vi "Pack Subscription Request.vi"(8 "error in (no error)":errorcluster, 9 "Subscription Policy":T1, 10 "Type":variant, 11 "Datum Name":string) -> (0 "error out":errorcluster, 3 "SubscriptionRequest":refnum<class "SubscriptionRequest.lvclass">)   [LabVIEW 2017, in "IMediator.lvlib" / "SubscriptionRequest.lvclass"]
doc: "<License>\nCopyright © 2017 Composed Systems, LLC | All rights reserved\nwww.composed.io\n\nAuthor: Ethan Stern <ethan.stern@composed.io>\n\nThis software is provided \"AS IS\" WITHOUT WARRANTIES, either express or implied, AND IS FOR EDUCATIONAL PURPOSES ONLY.\n</License>"
uses:
  <vilib>/gpm_packages/@cs/mva-core/Source/IMediator/SubscriptionRequest/SubscriptionRequest.lvclass
  <vilib>/gpm_packages/@cs/mva-core/Source/IMediator/ISubscriptionPolicy/ISubscriptionPolicy Reference.ctl
  <vilib>/gpm_packages/@cs/mva-core/Source/IMediator/ISubscriptionPolicy/ISubscriptionPolicy.lvclass
  <vilib>/gpm_packages/@cs/mva-core/Source/IMediator/SubscriptionRequest/SubscriptionRequest.lvclass/SubscriptionRequest.ctl
  <vilib>/Utility/error.llb/Error Cluster From Error Code.vi
  <vilib>/ErrorRing/Error Ring.xnode
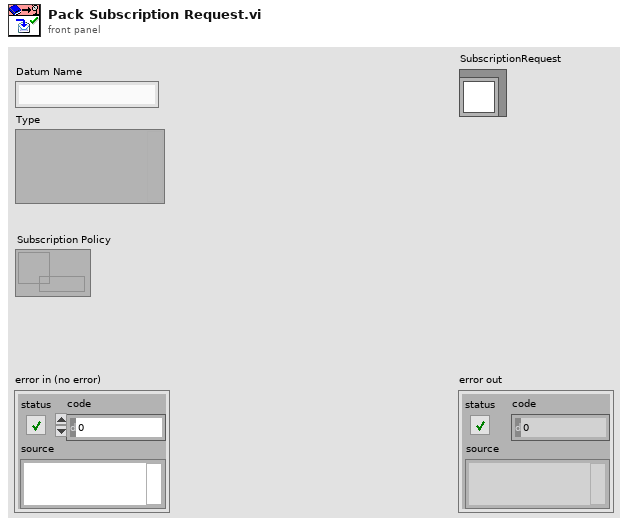
[diagram p1: front panel]
types:
  T1 = typedef "IMediator.lvlib/ISubscriptionPolicy.lvclass/ISubscriptionPolicy Reference.ctl" = refnum<data-value>
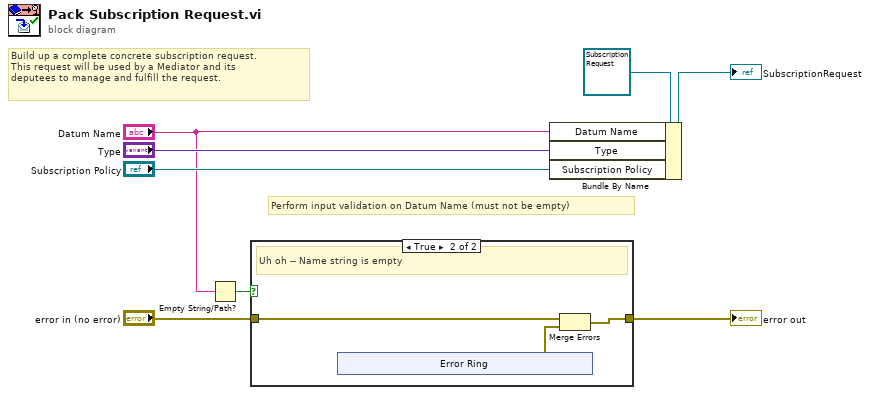
[diagram p0: block diagram]
diagram:
  # "Perform input validation on Datum Name (must not be empty)"
  # "Build up a complete concrete subscription request.\nThis request will be used by a Mediator and its\ndeputees to manage and fulfill the request."
  n1 = Empty String/Path?(string/path="Datum Name") -> (empty?=w4:bool)
  n2 = case shown="True" w4 {
    tunnel: "error in (no error)" -> [w9 w12]
    tunnel: [w9 w11] -> w2
    frame False {
      # "No problem!"
    }
    frame True {
      # "Uh oh -- Name string is empty"
      n3 = xnode "Error Ring"() -> ("error out"=w10:errorcluster)
      n4 = Merge Errors(w12, w10) -> (w11:errorcluster)
    }
  }
  "error out" <- w2
  n5 = Bundle By Name(cluster=refnum<class "SubscriptionRequest.lvclass"> refnum ("SubscriptionRequest in"), "Datum Name"="Datum Name", "Type"="Type", "Subscription Policy"="Subscription Policy") -> (→"SubscriptionRequest":refnum<class "SubscriptionRequest.lvclass">)
